vi "Calculate Mean Free Path.vi"(8 "error in (no error)":errorcluster, 11 "Air in":refnum<class "Air.lvclass">) -> (0 "error out":errorcluster, 2 "l (mm)":dbl, 3 "Air out":refnum<class "Air.lvclass">)   [LabVIEW 2015, in "Air.lvclass"]
uses:
  Air.lvclass
  Gas Properties.lvclass/Gas Properties.ctl
  Accessors/Read T (K).vi
  Accessors/Read P (mb).vi
  Atmospheric Constants.vi
  Atmospheric Library.lvlib
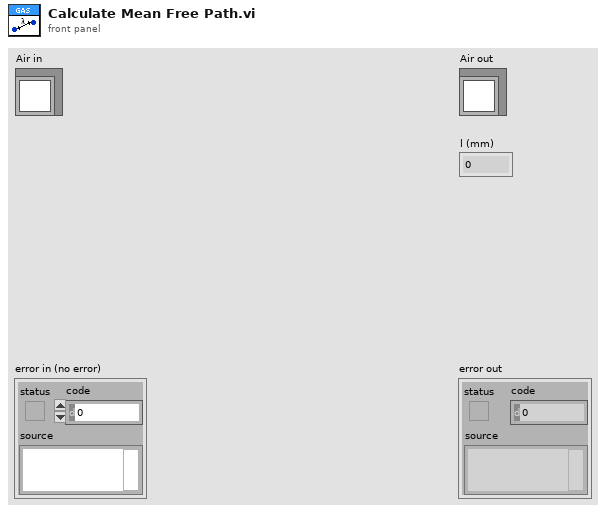
[diagram p1: front panel]
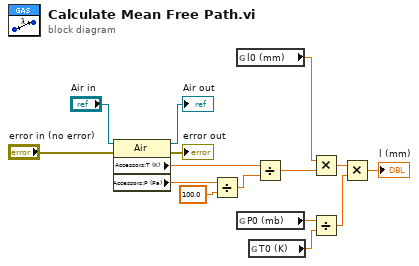
[diagram p0: block diagram]
diagram:
  n1 = property class="Air"(reference="Air in", error in="error in (no error)") -> (reference out=→"Air out":refnum<class "Air.lvclass">, error out=→"error out":errorcluster, "Accessors:T (K)"=w5:dbl, "Accessors:P (Pa)"=w6:dbl)
  n2 = Divide(x=w6, y=100.0) -> (x/y=w7:dbl)
  n3 = global read "Atmospheric Constants.vi" "l0 (mm)"() -> (w12:dbl)
  n4 = global read "Atmospheric Constants.vi" "P0 (mb)"() -> (w15:sgl)
  n5 = global read "Atmospheric Constants.vi" "T0 (K)"() -> (w14:sgl)
  n6 = Divide(x=w5, y=w7) -> (x/y=w13:dbl)
  n7 = Multiply(x=w12, y=w13) -> (x*y=w11:dbl)
  n8 = Divide(x=w15, y=w14) -> (x/y=w10:sgl)
  n9 = Multiply(x=w11, y=w10) -> (x*y=→"l (mm)":dbl)
